vi "CAM_ID_Request.vi"(11 "input cluster":T1={"Pinch-valve"="Test Sample", "XLP 6000 Pump"="MRJ", "Camera1"="", "Camera2"="", "Img_Capt"=FALSE, "Actuator"=FALSE, "Pump"=FALSE, "Cam 1"=FALSE, "Cam 2"=FALSE, "Empty_Refill"=FALSE, "Crop"=FALSE, "Light intensity"=0, "Exposure Time"=0.0, "Sample Name"="", "Operator"="", "Calibration 1"=path "C:/Users/au540322/Desktop/IHS_Project/images/Debris/Debris_0/Debris_0_2019_06_01-23-32-49-686.PNG", "Calibration 2"=path "C:/Users/au540322/Desktop/IHS_Project/images/Debris/Debris_0/Debris_0_2019_06_01-23-32-49-686.PNG", "Framerate"=100, "Timeout Sample"=500, "Collection date"="", "Sample size threshold"=500, "Empty start"=500, "Command"="", "Station"="", "Species Name"="", "Other Notes"="", "Aperture"=enum."Item 3", "Image Process Queue Size"=100, "Image Save Queue Size"=0, "Overload threshold"=0, "Max Framerate"=0, "Rectangle 1"={"Left"=0, "Top"=0, "Right"=0, "Bottom"=0, "Rotation"=0.0}, "Rectangle 2"={"Left"=0, "Top"=100, "Right"=100, "Bottom"=0, "Rotation"=0.0}, "Detection Region %"=200.0, "Detect 1"=path "C:/Users/au540322/Desktop/IHS_Project/images/Debris/Debris_0/Debris_0_2019_06_01-23-32-49-686.PNG", "Detect 2"=path "C:/Users/au540322/Desktop/IHS_Project/images/Debris/Debris_0/Debris_0_2019_06_01-23-32-49-686.PNG", "Max large object threshold"=500, "Open(T)/Close(F)"=FALSE, "Img_Capt Begin"=FALSE, "Dispense Speed"=0, "Flush Size"=0, "Location"="", "Latitude"="", "Longitude"="", "Determiner"="", "Sex"="", "Camera1_Img"=refnum, "Camera2_Img"=refnum, "Img1_Orig_Disp"=refnum, "Img2_Orig_Disp"=refnum, "Img1_Orig_RGB"=refnum, "Img2_Orig_RGB"=refnum, "Blue_Plane_Extract"=refnum, "Subtracted_Plane"=refnum, "Img1_Binary"=refnum, "Img2_Binary"=refnum, "Crop_Mask"=refnum, "Img1_Save"=refnum, "Img2_Save"=refnum, "Img1_Cali_Full"=refnum, "Img2_Cali_Full"=refnum, "Img1_Cali_Detect"=refnum, "Img2_Cali_Detect"=refnum, "Cam 1 queue"=refnum, "Cam 2 queue"=refnum, "Cam 1 - save queue"=refnum, "Cam 2 - save queue"=refnum, "Overlay_Ring"=0, "SystemVersion"=0, "System Serial"="", "Legacy Cam Attributes"=FALSE, "Camera Orientation 1"="", "Camera Orientation 2"="", "Pixel to mm 1"=0.0, "Pixel to mm 2"=0.0, "CAM1 Model"=enum."a2A5328-15ucBAS", "CAM2 Model"=enum."a2A5328-15ucBAS", "Flush Insect"=FALSE, "Pump Size"=FALSE, "Barcode"="", "Phase3"=FALSE, "Mega F3"="", "Container nr."=0.0, "Flush Error"=TRUE, "Start System"=FALSE, "Size Interval"=0.0, "Mun. of containers"=0.0, "Sorting sys."=FALSE, "Initial size"=0.0} {"SystemVersion" items=["Standard", "XL"]; "Overlay_Ring" items=["Session Data", "Extended Setup", "Buffer", "Camera", "Dispenser", "Stats", "Connections"]; "Flush Size" min=1; "Dispense Speed" min=1; "Rectangle 2"."Rotation" format="%.2f"; "Rectangle 2"."Left" scale=0.0..1024.0; "Rectangle 2"."Right" scale=0.0..1024.0; "Rectangle 1"."Rotation" format="%.2f"; "Rectangle 1"."Left" scale=0.0..1024.0; "Rectangle 1"."Right" scale=0.0..1024.0; "Max Framerate" min=1; "Overload threshold" min=1; "Image Save Queue Size" min=1; "Image Process Queue Size" min=1; "Empty start" min=1; "Sample size threshold" min=1; "Framerate" min=1; "Light intensity" scale=0.0..100.0}) -> (0 "error out":errorcluster, 2 "Connection?":bool, 3 "CAM_ID":T5)   [LabVIEW 2024]
uses:
  CAM_ID.ctl
  controls/Data.ctl
  <vilib>/userDefined/High Color/IMAQdx.ctl
  <vilib>/vision/Image Controls.llb/IMAQ Image.ctl
  b837ba4e-b16b-417a-9883-b1a8d73ee6f2.vi
panel:
  out "read buffer":string
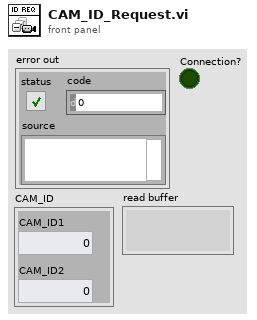
[diagram p1: front panel]
types:
  T1 = typedef "Data.ctl" = cluster{"Pinch-valve":refnum<visa-resource-name>, "XLP 6000 Pump":refnum<visa-resource-name>, "Camera1":T2, "Camera2":T2, "Img_Capt":bool, "Actuator":bool, "Pump":bool, "Cam 1":bool, "Cam 2":bool, "Empty_Refill":bool, "Crop":bool, "Light intensity":i32, "Exposure Time":dbl, "Sample Name":string, "Operator":string, "Calibration 1":path, "Calibration 2":path, "Framerate":i32, "Timeout Sample":i32, "Collection date":string, "Sample size threshold":i32, "Empty start":u32, "Command":string, "Station":string, "Species Name":string, "Other Notes":string, "Aperture":enum32{"Item 0", "Item 1", "Item 2", "Item 3"}, "Image Process Queue Size":i32, "Image Save Queue Size":i32, "Overload threshold":i32, "Max Framerate":i32, "Rectangle 1":T3, "Rectangle 2":T3, "Detection Region %":dbl, "Detect 1":path, "Detect 2":path, "Max large object threshold":i32, "Open(T)/Close(F)":bool, "Img_Capt Begin":bool, "Dispense Speed":i32, "Flush Size":i32, "Location":string, "Latitude":string, "Longitude":string, "Determiner":string, "Sex":string, "Camera1_Img":T4, "Camera2_Img":T4, "Img1_Orig_Disp":T4, "Img2_Orig_Disp":T4, "Img1_Orig_RGB":T4, "Img2_Orig_RGB":T4, "Blue_Plane_Extract":T4, "Subtracted_Plane":T4, "Img1_Binary":T4, "Img2_Binary":T4, "Crop_Mask":T4, "Img1_Save":T4, "Img2_Save":T4, "Img1_Cali_Full":T4, "Img2_Cali_Full":T4, "Img1_Cali_Detect":T4, "Img2_Cali_Detect":T4, "Cam 1 queue":refnum<queue>, "Cam 2 queue":refnum<queue>, "Cam 1 - save queue":refnum<queue>, "Cam 2 - save queue":refnum<queue>, "Overlay_Ring":u16, "SystemVersion":u16, "System Serial":string, "Legacy Cam Attributes":bool, "Camera Orientation 1":string, "Camera Orientation 2":string, "Pixel to mm 1":dbl, "Pixel to mm 2":dbl, "CAM1 Model":enum16{"a2A5328-15ucBAS", "acA1920-155uc"}, "CAM2 Model":enum16{"a2A5328-15ucBAS", "acA1920-155uc"}, "Flush Insect":bool, "Pump Size":bool, "Barcode":string, "Phase3":bool, "Mega F3":refnum<visa-resource-name>, "Container nr.":dbl, "Flush Error":bool, "Start System":bool, "Size Interval":dbl, "Mun. of containers":dbl, "Sorting sys.":bool, "Initial size":dbl}
  T2 = typedef "IMAQdx.ctl" = refnum<k21>
  T3 = typedef "IMAQ Rectangle" = cluster{"Left":i32, "Top":i32, "Right":i32, "Bottom":i32, "Rotation":dbl}
  T4 = typedef "IMAQ Image.ctl" = refnum<image>
  T5 = typedef "CAM_ID.ctl" = cluster{"CAM_ID1":i32, "CAM_ID2":i32}
  T6 = cluster{"[0]":i32, "[1]":i32, "[2]":i32, "[3]":i32, "[4]":i32, "[5]":i32, "[6]":i32, "[7]":i32, "[8]":i32}
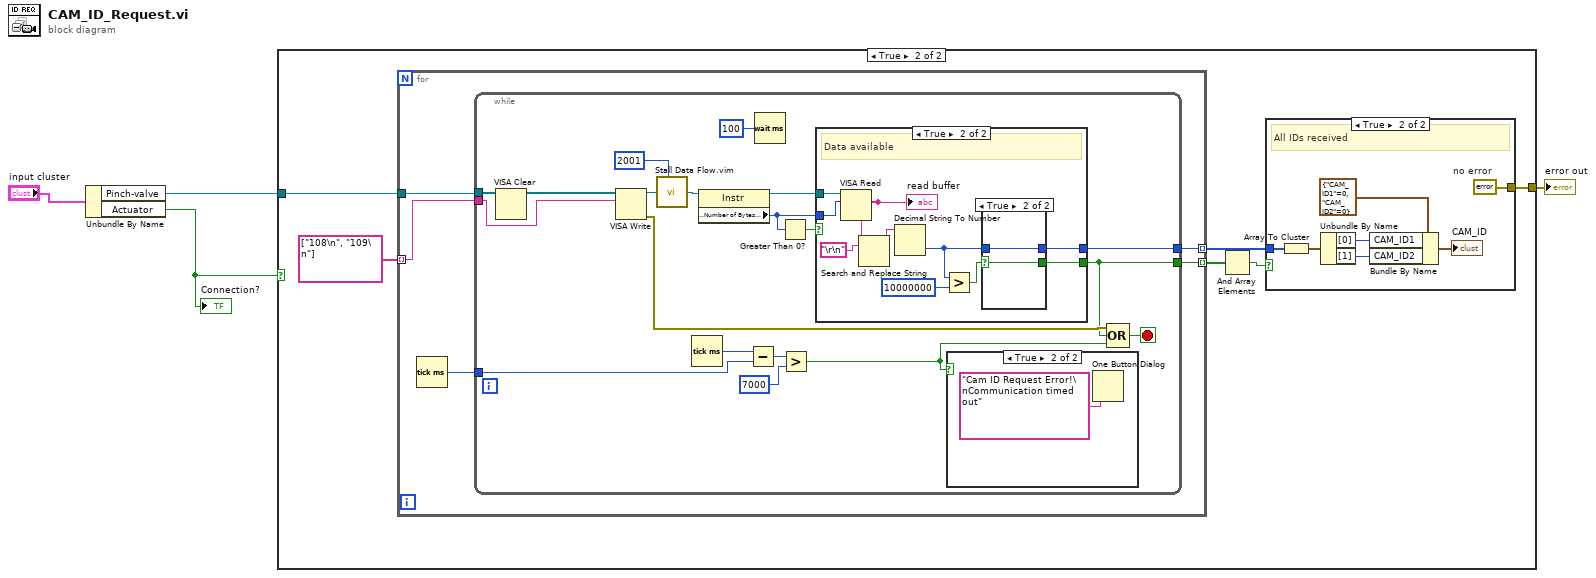
[diagram p0: block diagram]
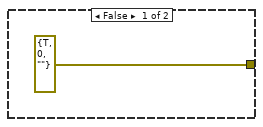
[diagram p2: hidden frame]
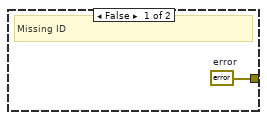
[diagram p3: hidden frame]
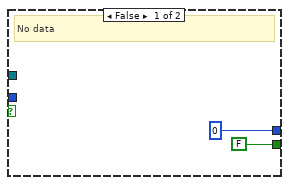
[diagram p5: hidden frame]
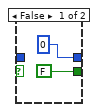
[diagram p6: hidden frame]
diagram:
  n1 = Unbundle By Name("input cluster") -> ("Pinch-valve"=w2:refnum<visa-resource-name>, "Actuator"=w1:bool)
  "Connection?" <- w1
  n2 = case shown="True" w1 {
    tunnel: [errorcluster {"status"=TRUE, "code"=0, "source"=""} ("error") w8] -> w4
    tunnel: w2 -> [_ w7]
    frame False {
    }
    frame True {
      n3 = for {
        tunnel: w7 -> [w20]
        tunnel: string[] ["108\n", "109\n"] -> [w21] mode=indexing
        tunnel: [w24] -> w9 mode=indexing
        tunnel: [w23] -> w11 mode=indexing
        n4 = Tick Count (ms)() -> (millisecond timer value=w22:u32)
        n5 = while {
          tunnel: [w43] -> w24
          tunnel: [w29] -> w23
          tunnel: w22 -> [w35]
          tunnel: w21 -> [w25]
          tunnel: w20 -> [w32]
          stop <- w40 stop-if-true
          n6 = VISA Clear(VISA resource name=w32) -> (VISA resource name out=w28:refnum<visa-resource-name>)  [unwired: 1 in, 1 out]
          n7 = VISA Write(VISA resource name=w28, write buffer=w25) -> (VISA resource name out=w33:refnum<visa-resource-name>, error out=w30:errorcluster)  [unwired: 1 in, 1 out]
          n8 = call "Stall Data Flow.vim"("value in"=w33, "milliseconds to wait"=u32 2001) -> ("value out"=w31:refnum<visa-resource-name>)  [unwired: 1 out]
          n9 = Tick Count (ms)() -> (millisecond timer value=w37:u32)
          n10 = property class="Instr"(reference=w31) -> (reference out=w26:refnum<visa-resource-name>, "Serial Settings:Number of Bytes at Serial Port"=w42:u32)  [unwired: 1 in, 1 out]
          n11 = Subtract(x=w37, y=w35) -> (x-y=w38:u32)
          n12 = Wait (ms)(milliseconds to wait=u32 100) -> ()  [unwired: 1 out]
          n13 = Greater Than 0?(x=w42) -> (x > 0?=w39:bool)
          n14 = Greater?(x=w38, y=u32 7000 ("x")) -> (0:w34:bool)
          n15 = case shown="True" w39 {
            tunnel: w42 -> [_ w56]
            tunnel: w26 -> [_ w55]
            tunnel: [0 w50] -> w43
            tunnel: [FALSE w49] -> w29
            frame False {
              # "No data"
            }
            frame True {
              # "Data available"
              n16 = VISA Read(VISA resource name=w55, byte count=w56) -> (read buffer=w54:string)  [unwired: 1 in, 3 out]
              "read buffer" <- w54
              n17 = Search and Replace String(input string=w54, search string="\r\n") -> (result string=w48:string)  [unwired: 6 in, 3 out]
              n18 = Decimal String To Number(string=w48) -> (number=w51:i32)  [unwired: 2 in, 1 out]
              n19 = Greater?(x=w51, y=10000000) -> (0:w52:bool)
              n20 = case shown="True" w52 {
                selector: w52 -> [_ w59]
                tunnel: [0 w60] -> w50
                tunnel: w51 -> [_ w60]
                tunnel: [FALSE w59] -> w49
                frame False {
                }
                frame True {
                }
              }
            }
          }
          n21 = case shown="True" w34 {
            frame False {
            }
            frame True {
              n22 = One Button Dialog(message="Cam ID Request Error!\nCommunication timed out") -> ()  [unwired: 1 in, 1 out]
            }
          }
          n23 = Compound Arithmetic op=OR(w30, w29, w34) -> (w40:bool)
        }
      }
      n24 = And Array Elements(Boolean array=w11) -> (logical AND=w10:bool)
      n25 = case shown="True" w10 {
        tunnel: w9 -> [_ w14]
        tunnel: [w12 w13] -> w8
        frame False {
          w12 = errorcluster {"status"=TRUE, "code"=0, "source"=""}  # error
          # "Missing ID"
        }
        frame True {
          w13 = errorcluster {"status"=FALSE, "code"=0, "source"=""}  # no error
          # "All IDs received"
          n26 = Array To Cluster(array=w14) -> (cluster=w16:T6)
          n27 = Unbundle By Name(w16) -> ("[0]"=w18:i32, "[1]"=w19:i32)
          n28 = Bundle By Name(cluster=T5 {"CAM_ID1"=0, "CAM_ID2"=0} ("CAM_ID 2"), "CAM_ID1"=w18, "CAM_ID2"=w19) -> (→"CAM_ID":T5)
        }
      }
    }
  }
  "error out" <- w4
